vi "Receipt.vi"(9 "Account Number":string, 10 "Value":string, 11 "Operation":string) -> (2 "Output":string)   [LabVIEW 2023]
panel:
  out "date/time string":string
  out "current time":timestamp
  # "Input"
  # "Auto-generated Content"
  # "Errors"
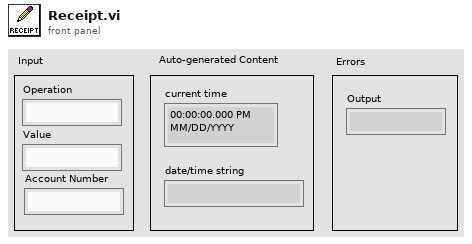
[diagram p1: front panel]
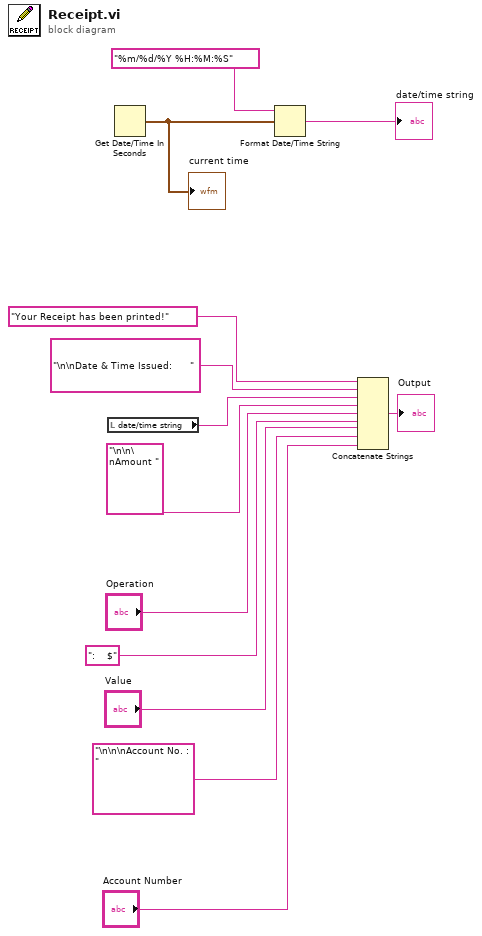
[diagram p0: block diagram]
diagram:
  n1 = local read "date/time string"() -> (w10:string)
  n2 = Get Date/Time In Seconds() -> (seconds since 1Jan1904=w13:timestamp)
  "current time" <- w13
  n3 = Format Date/Time String(time format string (%c)="%m/%d/%Y %H:%M:%S", seconds (now)=w13) -> (date/time string=→"date/time string":string)  [unwired: 1 in]
  n4 = Concatenate Strings("Your Receipt has been printed!" ("string"), "\n\nDate & Time Issued:      " ("string"), w10, "\n\n\nAmount " ("string"), "Operation", ":    $" ("string"), "Value", "\n\n\nAccount No. :    " ("string"), "Account Number") -> (→"Output":string)
